vi "Oriantation Process.vi"   [LabVIEW 2013]
uses:
  Oritentation Global.vi
types:
  T1 = cluster{"Front Right Reads":dbl, "Front Left Reads ":dbl, "Rear Reads":dbl, "Camera Mounted Reads":dbl, "Calculated Robot Angle":dbl, "Distance on Ground":dbl, "Front Right Distance":dbl, "Front Left Distance":dbl, "Rear Distance":dbl, "Camera Mounted Distance":dbl}
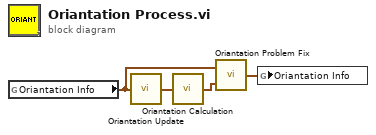
[diagram p0: block diagram]
diagram:
  n1 = global read "Oritentation Global.vi" "Oriantation Info"() -> (w2:T1)
  n2 = call "Oriantation Update.vi"("Oriantation Info In"=w2) -> ("Oriantation Info Out"=w3:T1)
  n3 = call "Oriantation Calculation.vi"("Oriantation Info In"=w3) -> ("Oriantation Info Out"=w4:T1)
  n4 = call "Oriantation Problem Fix.vi"("Oriantation Info Modified"=w4, "Oriantation Info Origianl"=w2) -> ("Oriantation Info Fixed"=w1:T1)
  n5 = global write "Oritentation Global.vi" "Oriantation Info"(w1) -> ()
